vi "PC_Daten von cRIO.vi"() -> (2 "LifeBit":bool)   [LabVIEW 2020, in "Kommunikation mit cRIO.lvlib"]
uses:
  Kommunikation mit cRIO.lvlib
  Allgemein/Aktionen Daten am cRIO speichern.ctl
  Aktionen FGV Druckregler.ctl
  PNS/Aktion FGV AO PNS.ctl
  Funktionstasten/Funktionstasten-Aktion.ctl
  Funktionstasten/Zustaende.ctl
  Allgemein/allgemeine Sub-VIs.lvlib
  PNS/PNS.lvlib
  Funktionstasten/Funktionstasten.lvlib
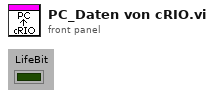
[diagram p1: front panel]
types:
  T1 = typedef "PNS.lvlib/Aktion FGV AO PNS.ctl" = enum16{"lesen", "schreiben"}
  T2 = typedef "Kommunikation mit cRIO.lvlib/Aktionen FGV Druckregler.ctl" = enum16{"lesen", "Parameter", "Istwerte", "laden", "speichern"}
  T3 = typedef "allgemeine Sub-VIs.lvlib/Aktionen Daten am cRIO speichern.ctl" = enum16{"lesen", "speichern setzen", "speichern reset", "gespeichert"}
  T4 = typedef "Funktionstasten.lvlib/Funktionstasten-Aktion.ctl" = enum16{"Initialisieren", "Zustand setzen", "Taste gedrückt", "Fehler speichern", "Lesen", "Manuell", "Remote", "Bitparallel", "Samplepoint", "Zeit Prüfen", "reset Umschalten"}
  T5 = typedef "Funktionstasten.lvlib/Zustaende.ctl" = enum16{"Standby", "Pause", "Eco", "Messen", "Kalibrieren", "Spülen Filter", "Spülen Leitung", "Umgebungsluft", "0-Gas", "Cal-Gas", "CG zu PNS", "-------------", "Init 1", "Init 2", "Init 3", "Init 4", "Messen vorbereiten", "Messen durchführen", "Exit"}
  T6 = cluster{"Array[0]":sgl, "Array[1]":sgl, "Array[2]":sgl, "Array[3]":sgl, "Array[4]":sgl, "Array[5]":sgl, "Array[6]":sgl, "Array[7]":sgl, "Array[8]":sgl, "Array[9]":sgl, "Array[10]":sgl, "Array[11]":sgl}
  T7 = cluster{"Array[0]":sgl, "Array[1]":sgl, "Array[2]":sgl, "Array[3]":sgl, "Array[4]":sgl, "Array[5]":sgl, "Array[6]":sgl, "Array[7]":sgl, "Array[8]":sgl, "Array[9]":sgl, "Array[10]":sgl, "Array[11]":sgl, "Array[12]":sgl, "Array[13]":sgl, "Array[14]":sgl, "Array[15]":sgl, "Array[16]":sgl}
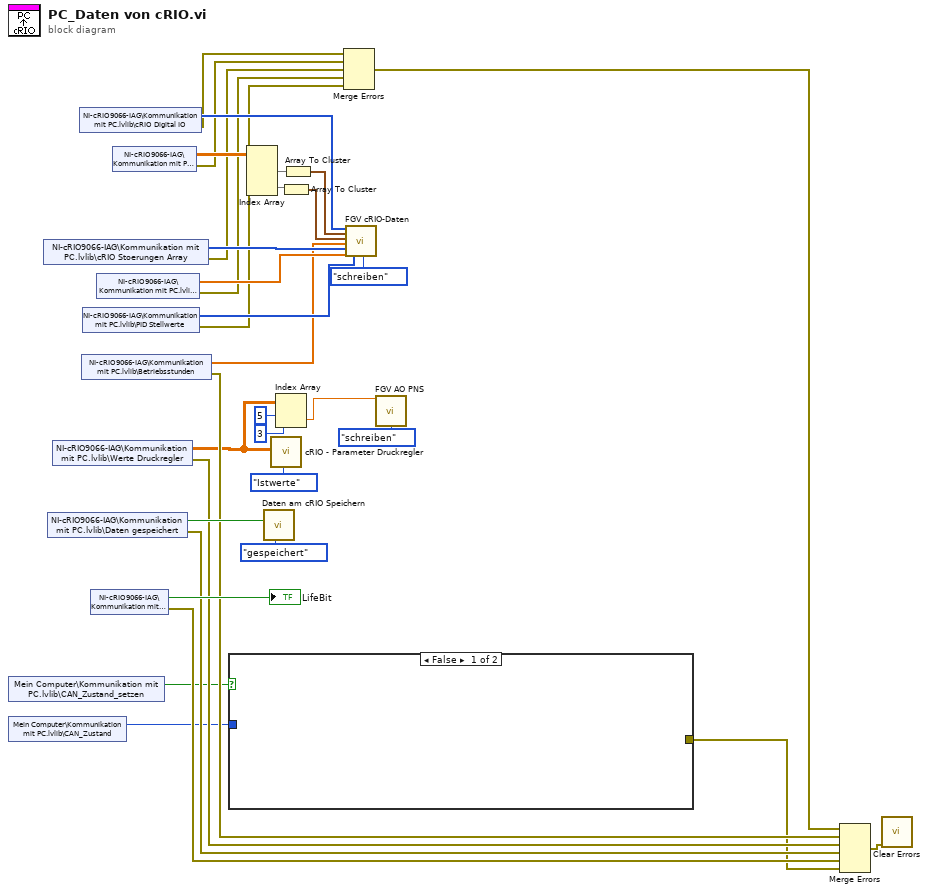
[diagram p0: block diagram]
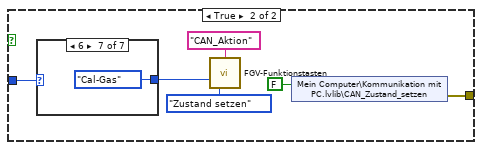
[diagram p2: hidden frame]
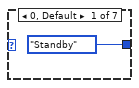
[diagram p3: hidden frame]
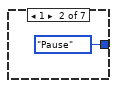
[diagram p4: hidden frame]
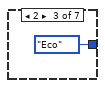
[diagram p5: hidden frame]
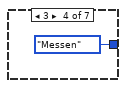
[diagram p6: hidden frame]
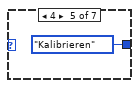
[diagram p7: hidden frame]
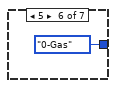
[diagram p8: hidden frame]
diagram:
  n1 = shared-variable "Mein Computer\\Kommunikation mit PC.lvlib\\CAN_Zustand_setzen"() -> (w3:bool)  [unwired: 1 in, 1 out]
  n2 = shared-variable "Mein Computer\\Kommunikation mit PC.lvlib\\CAN_Zustand"() -> (w1:u16)  [unwired: 1 in, 1 out]
  n3 = shared-variable "NI-cRIO9066-IAG\\Kommunikation mit PC.lvlib\\cRIO Stoerungen Array"() -> (w34:u64[], error out=w21:errorcluster)  [unwired: 1 in]
  n4 = shared-variable "NI-cRIO9066-IAG\\Kommunikation mit PC.lvlib\\Daten gespeichert"() -> (w32:bool, error out=w15:errorcluster)  [unwired: 1 in]
  n5 = shared-variable "NI-cRIO9066-IAG\\Kommunikation mit PC.lvlib\\Werte Druckregler"() -> (w7:sgl[][], error out=w16:errorcluster)  [unwired: 1 in]
  n6 = shared-variable "NI-cRIO9066-IAG\\Kommunikation mit PC.lvlib\\cRIO Digital IO"() -> (w30:u32[], error out=w23:errorcluster)  [unwired: 1 in]
  n7 = shared-variable "NI-cRIO9066-IAG\\Kommunikation mit PC.lvlib\\Betriebsstunden"() -> (w13:dbl[], error out=w18:errorcluster)  [unwired: 1 in]
  n8 = shared-variable "NI-cRIO9066-IAG\\Kommunikation mit PC.lvlib\\PID Stellwerte"() -> (w25:i16[], error out=w19:errorcluster)  [unwired: 1 in]
  n9 = shared-variable "NI-cRIO9066-IAG\\Kommunikation mit PC.lvlib\\LifeBit"() -> (→"LifeBit":bool, error out=w14:errorcluster)  [unwired: 1 in]
  n10 = shared-variable "NI-cRIO9066-IAG\\Kommunikation mit PC.lvlib\\CPU Status"() -> (w29:sgl[], error out=w20:errorcluster)  [unwired: 1 in]
  n11 = shared-variable "NI-cRIO9066-IAG\\Kommunikation mit PC.lvlib\\cRIO AI"() -> (w28:sgl[][], error out=w22:errorcluster)  [unwired: 1 in]
  n12 = case shown="False" w3 {
    tunnel: [_ w40] -> w2
    tunnel: w1 -> [_ w39]
    frame False {
    }
    frame True {
      n13 = case shown="6" w39 {
        tunnel: [Zustaende."Standby" ("Zustand") Zustaende."Pause" ("Zustand") Zustaende."Eco" ("Zustand") Zustaende."Messen" ("Zustand") Zustaende."Kalibrieren" ("Zustand") Zustaende."0-Gas" ("Zustand") Zustaende."Cal-Gas" ("Zustand")] -> w36
        frame 0, Default {
        }
        frame 1 {
        }
        frame 2 {
        }
        frame 3 {
        }
        frame 4 {
        }
        frame 5 {
        }
        frame 6 {
        }
      }
      n14 = call "FGV-Funktionstasten.vi"("Herkunft"="CAN_Aktion", "Zustand"=w36, "Aktion"=Funktionstasten-Aktion."Zustand setzen") -> ()  [unwired: 5 in, 8 out]
      n15 = shared-variable "Mein Computer\\Kommunikation mit PC.lvlib\\CAN_Zustand_setzen"(FALSE ("CAN_Zustand_setzen")) -> (error out=w40:errorcluster)  [unwired: 1 in]
    }
  }
  n16 = Index Array(array=w28) -> (element #1=w11:sgl[], element #2=w10:sgl[])  [unwired: 4 in]
  n17 = call "Daten am cRIO Speichern.vi"("Aktionen"=Aktionen_Daten_am_cRIO_speichern."gespeichert", "gespeichert"=w32) -> ()  [unwired: 8 in, 2 out]
  n18 = call "cRIO - Parameter Druckregler.vi"("Istwerte Regler"=w7, "Aktion"=Aktionen_FGV_Druckregler."Istwerte") -> ()  [unwired: 8 in, 10 out]
  n19 = Index Array(array=w7, index (row)=5 ("Index (Zeile)"), index (col)=3 ("Deaktivierter Index (Spalte)")) -> (element=w4:sgl)
  n20 = Array To Cluster(array=w10) -> (cluster=w9:T6)
  n21 = Array To Cluster(array=w11) -> (cluster=w27:T7)
  n22 = Merge Errors(w23, w22, w21, w20, w19) -> (w12:errorcluster)
  n23 = call "FGV cRIO-Daten.vi"("cRIO DI - DO"=w30, "Analog Input"=w27, "TC Eingänge"=w9, "Stickstoff Befüllung"=w13, "Störungen"=w34, "CPU Status"=w29, "PID Stellwerte"=w25, "Aktion"=enum16{"lesen", "schreiben"}."schreiben") -> ()  [unwired: 2 in, 10 out]
  n24 = call "FGV AO PNS.vi"("AO PROP"=w4, "Aktion"=Aktion_FGV_AO_PNS."schreiben") -> ()  [unwired: 12 in, 2 out]
  n25 = Merge Errors(w12, w18, w16, w15, w14, w2) -> (w17:errorcluster)
  n26 = call <vilib>:"Clear Errors.vi"("error in (no error)"=w17) -> ()  [unwired: 5 in, 2 out]
